vi "Read_DevState.vi"(8 "error in (no error)":errorcluster, 11 "Multiplexer_Opmux in":refnum<class "Multiplexer_Opmux.lvclass">) -> (0 "error out":errorcluster, 2 "DevState":bool, 3 "Multiplexer_Opmux out":refnum<class "Multiplexer_Opmux.lvclass">)   [LabVIEW 2014, in "Multiplexer_Opmux.lvclass"]
uses:
  Multiplexer_Opmux.lvclass
  Multiplexer_Opmux.lvclass/Multiplexer_Opmux.ctl
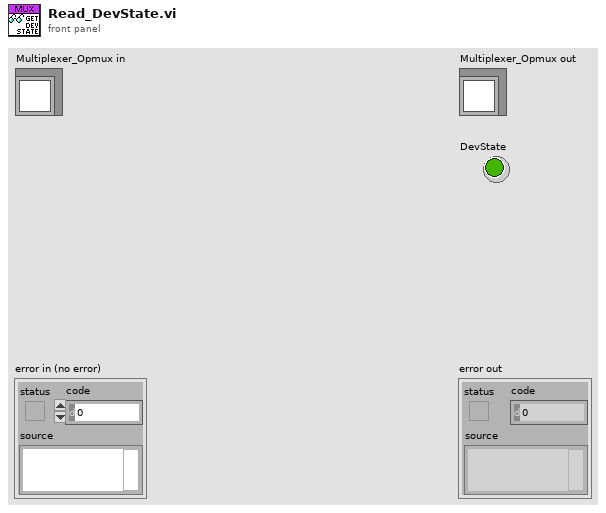
[diagram p1: front panel]
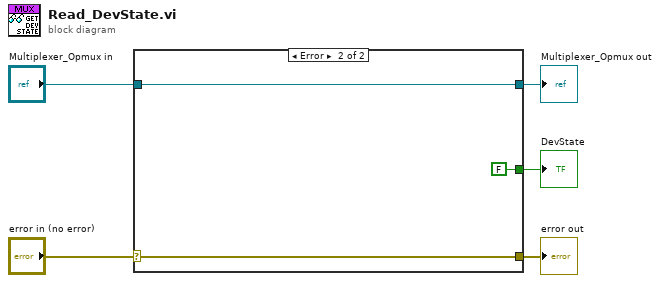
[diagram p0: block diagram]
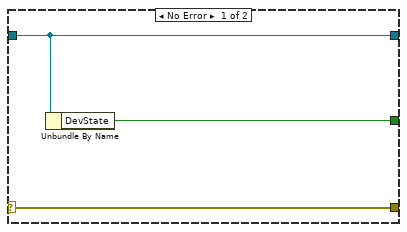
[diagram p2: hidden frame]
diagram:
  n1 = case shown="Error" "error in (no error)" {
    selector: "error in (no error)" -> [w8 w10]
    tunnel: [w8 w10] -> w4
    tunnel: [w7 w11] -> w2
    tunnel: "Multiplexer_Opmux in" -> [w7 w11]
    tunnel: [w6 FALSE ("DevState")] -> w1
    frame No Error {
      n2 = Unbundle By Name(w7) -> ("DevState"=w6:bool)
    }
    frame Error {
    }
  }
  "error out" <- w4
  "Multiplexer_Opmux out" <- w2
  "DevState" <- w1
